vi "Omron TCP FINS-Initialize.vi"(8 "error in":errorcluster, 11 "Connection Data In":T3={"Server IP Address"="", "Client IP Address"="", "Port"=0, "Timeout"=60000, "Unit Number"=0}) -> (0 "error out":errorcluster, 3 "Buffer Data":T1)   [LabVIEW 2016]
uses:
  Data Def/Omron TCP FINS-Connection Data.ctl
  Data Def/Omron TCP FINS-Buffer Data.ctl
  Data Def/Omron TCP FINS-Command Code.ctl
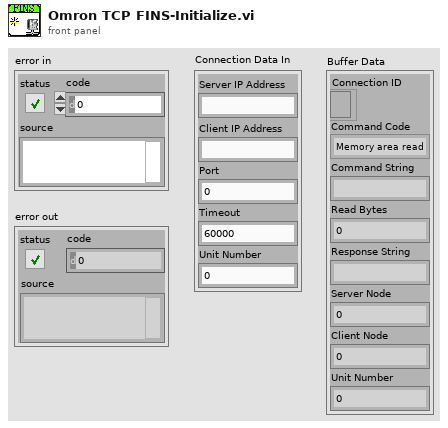
[diagram p1: front panel]
types:
  T1 = typedef "Omron TCP FINS-Buffer Data.ctl" = cluster{"Connection ID":refnum<k5>, "Command Code":T2, "Command String":string, "Read Bytes":i32, "Response String":string, "Server Node":u8, "Client Node":u8, "Unit Number":u8}
  T2 = typedef "Omron TCP FINS-Command Code.ctl" = enum16{"Memory area read", "Memory area write"}
  T3 = typedef "Omron TCP FINS-Connection Data.ctl" = cluster{"Server IP Address":string, "Client IP Address":string, "Port":u16, "Timeout":i32, "Unit Number":u8}
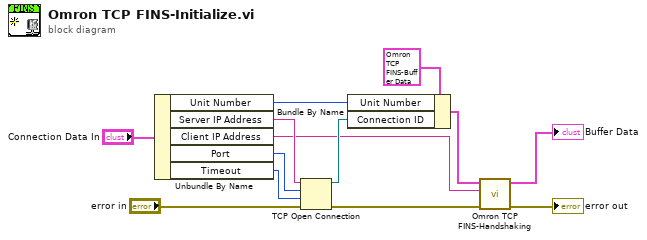
[diagram p0: block diagram]
diagram:
  n1 = Unbundle By Name("Connection Data In") -> ("Unit Number"=w4:u8, "Server IP Address"=w5:string, "Client IP Address"=w3:string, "Port"=w11:u16, "Timeout"=w10:i32)
  n2 = TCP Open Connection(address=w5, remote port or service name=w11, timeout ms (60000)=w10, error in (no error)="error in") -> (connection ID=w8:refnum<k5>, error out=w7:errorcluster)  [unwired: 1 in]
  n3 = Bundle By Name(cluster=T1 {"Connection ID"=refnum, "Command Code"=enum."Memory area read", "Command String"="", "Read Bytes"=0, "Response String"="", "Server Node"=0, "Client Node"=0, "Unit Number"=0} ("Buffer Data"), "Unit Number"=w4, "Connection ID"=w8) -> (w2:T1)
  n4 = call "Omron TCP FINS-Handshaking.vi"("error in"=w7, "Client IP"=w3, "Buffer Data In"=w2) -> ("error out"=→"error out":errorcluster, "Buffer Data Out"=→"Buffer Data":T1)  [unwired: 7 in]
